vi "rpr -- read write buttons.vi"(7 "what":enum16{"read", "none", "write"}(ring)=enum."write", 8 "appended array":refnum<vi>[](array[refnum]), 9 "peaks":i32[](array[numeric])=[572], 11 "9w folder path":path=path "C:/data/RUS/Experiment/ProbeTest/Probe10/YBCO_6/sweep2/9w") -> ()   [LabVIEW 2014]
uses:
  <vilib>/Utility/file.llb/Read From Spreadsheet File (string).vi
  <vilib>/Utility/file.llb/Write To Spreadsheet File (string).vi
  <vilib>/regexp/Match Regular Expression.xnode
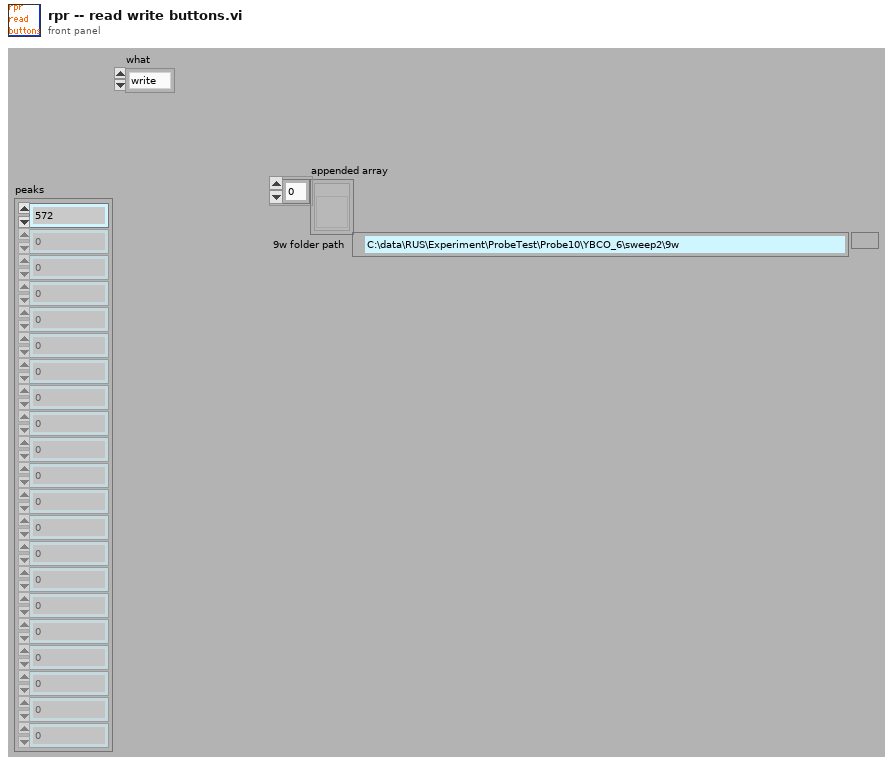
[diagram p1: front panel]
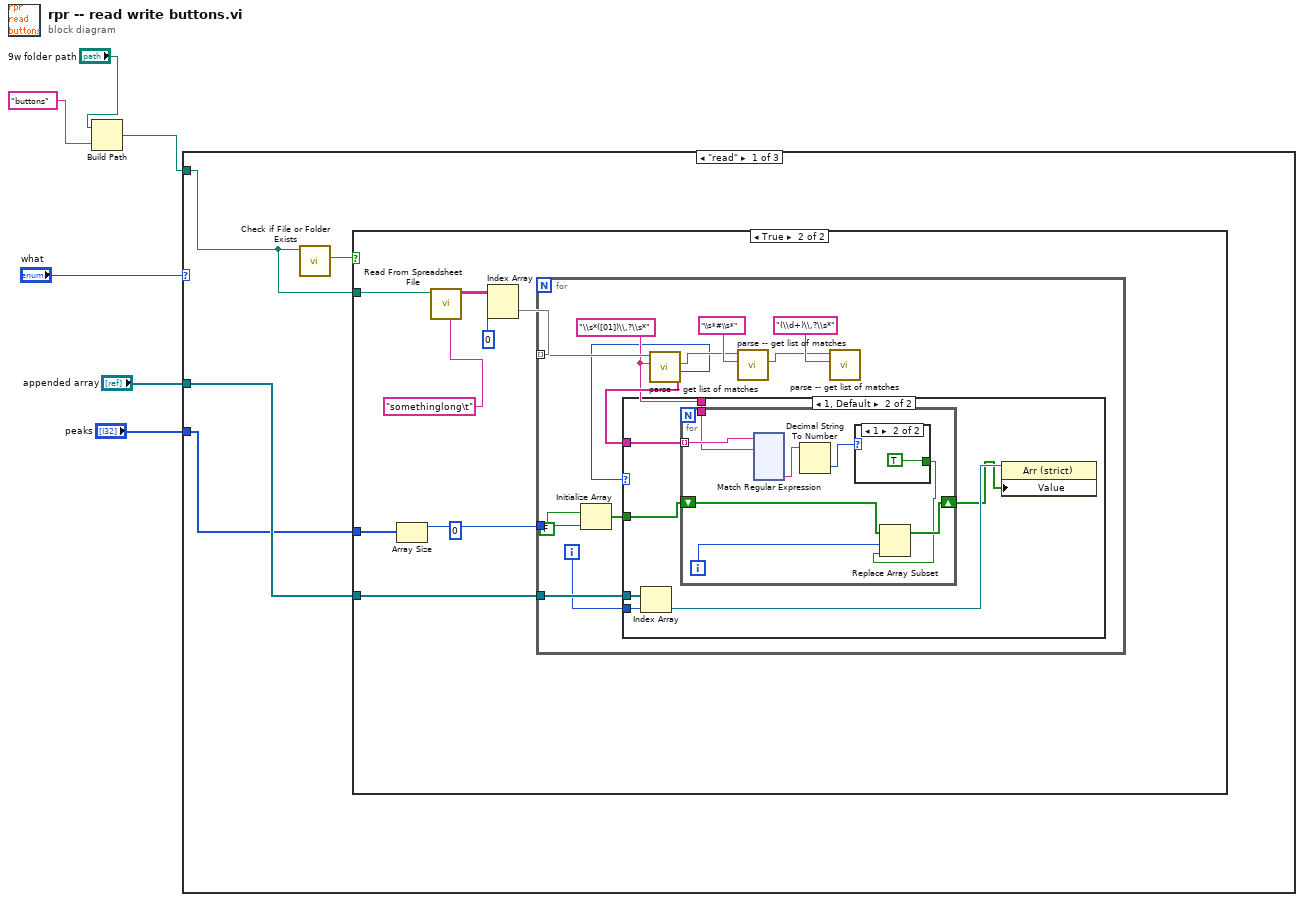
[diagram p0: block diagram]
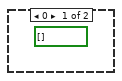
[diagram p3: hidden frame]
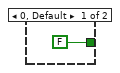
[diagram p4: hidden frame]
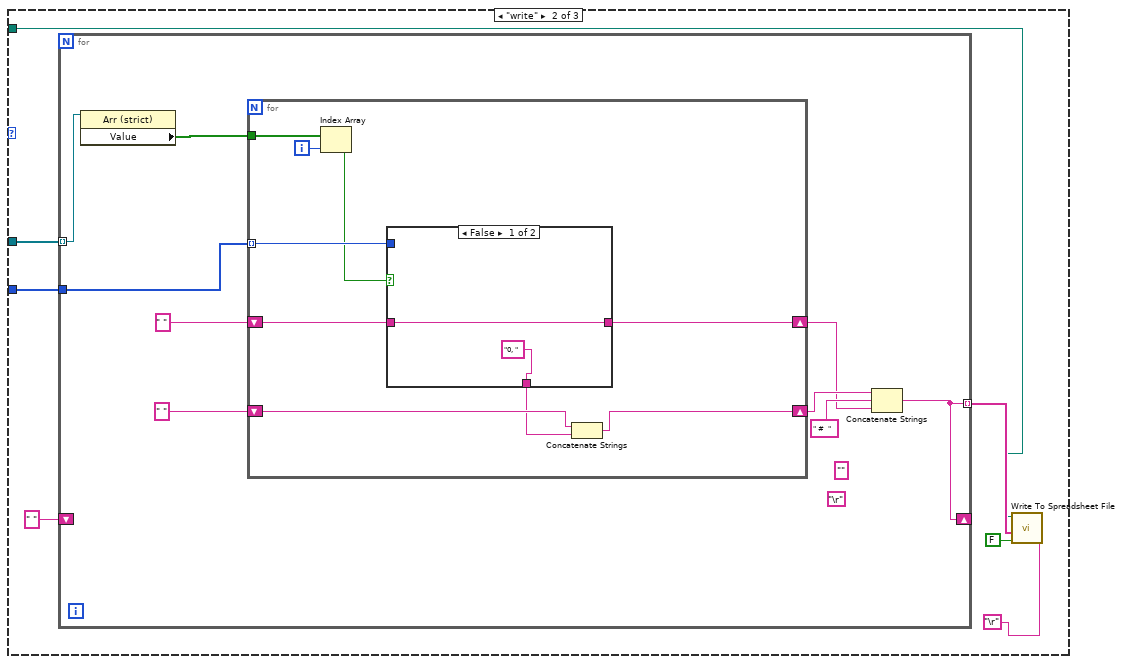
[diagram p5: hidden frame]
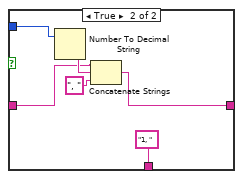
[diagram p6: hidden frame]
diagram:
  n1 = Build Path(base path="9w folder path", name or relative path="buttons") -> (appended path=w1:path)
  n2 = case shown="\"read\"" "what" {
    tunnel: "appended array" -> [w8 w168 _]
    tunnel: "peaks" -> [w7 w167 _]
    tunnel: w1 -> [w9 w162 _]
    frame "read" {
      n3 = call <vilib>:"Check if File or Folder Exists.vi"("path"=w9) -> ("file or folder exists?"=w10:bool)  [unwired: 8 in, 2 out]
      n4 = case shown="True" w10 {
        tunnel: w9 -> [_ w18]
        tunnel: w8 -> [_ w13]
        tunnel: w7 -> [_ w12]
        frame False {
        }
        frame True {
          (unwired) 0
          n5 = Array Size(array=w12) -> (size(s)=w11:i32)
          n6 = call-poly <vilib>:"Read From Spreadsheet File.vi"("delimiter (\\t)"="somethinglong\t" ("delimiter (\\t)"), "file path (dialog if empty)"=w18) -> ("all rows"=w16:string[][])  [unwired: 5 in, 4 out]
          n7 = Index Array(array=w16, index (col)=0) -> (element=w14:string[])  [unwired: 1 in]
          n8 = for {
            tunnel: w14 -> [w31] mode=indexing
            tunnel: w13 -> [w26]
            tunnel: w11 -> [w20]
            i -> [w25]
            w23 = "\\s*([01])\\,?\\s*" ("format string")
            n9 = Initialize Array(FALSE, w20) -> (w19:bool[])
            n10 = call "parse -- get list of matches.vi"("regexp"=w23, "string"=w31) -> ("Array"=w24:string[], "number of free elastic constants"=w22:i32, "after match"=w28:string)  [unwired: 7 in]
            n11 = case shown="1, Default" w22 {
              tunnel: w26 -> [_ w38]
              tunnel: w25 -> [_ w37]
              tunnel: w24 -> [_ w36]
              tunnel: w23 -> [_ w35]
              tunnel: w19 -> [_ w33]
              frame 0 {
                (unwired) bool[] []
              }
              frame 1, Default {
                n12 = Index Array(array=w38, index=w37) -> (element=w34:refnum<vi>)
                n13 = for {
                  tunnel: w36 -> [w46] mode=indexing
                  tunnel: w35 -> [w45]
                  shift-right: [w41] -> w32
                  shift-left: w33 -> [w42]
                  i -> [w40]
                  n14 = xnode "Match Regular Expression"("input string"=w46, "regular expression"=w45) -> ("submatch 1"=w44:string)  [unwired: 4 in, 5 out]
                  n15 = Decimal String To Number(string=w44) -> (number=w43:i32)  [unwired: 2 in, 1 out]
                  n16 = case shown="1" w43 {
                    tunnel: [FALSE TRUE] -> w39
                    frame 0, Default {
                    }
                    frame 1 {
                    }
                  }
                  n17 = Replace Array Subset(array=w42, new element=w39, index=w40) -> (w41:bool[])
                }
                n18 = property class="Arr (strict)"(reference=w34, "Value"=w32) -> ()  [unwired: 1 in, 2 out]
              }
            }
            n19 = call "parse -- get list of matches.vi"("regexp"="\\s*#\\s*" ("format string"), "string"=w28) -> ("after match"=w27:string)  [unwired: 7 in, 2 out]
            n20 = call "parse -- get list of matches.vi"("regexp"="(\\d+)\\,?\\s*" ("format string"), "string"=w27) -> ()  [unwired: 7 in, 3 out]
          }
        }
      }
    }
    frame "write" {
      n21 = for {
        tunnel: w168 -> [w177] mode=indexing
        tunnel: w167 -> [w175]
        shift-right: [w169] -> _
        shift-left: " " -> [_]
        tunnel: [w169] -> w165 mode=indexing
        (unwired) "\r"
        (unwired) ""
        n22 = property class="Arr (strict)"(reference=w177) -> ("Value"=w176:bool[])  [unwired: 1 in, 2 out]
        n23 = for {
          tunnel: w176 -> [w185]
          tunnel: w175 -> [w182] mode=indexing
          shift-right: [w183] -> w170
          shift-left: " " -> [w184]
          shift-right: [w178] -> w172
          shift-left: " " -> [w180]
          i -> [w186]
          n24 = Index Array(array=w185, index=w186) -> (element=w181:bool)
          n25 = case shown="False" w181 {
            tunnel: w184 -> [w188 w192]
            tunnel: [w188 w191] -> w183
            tunnel: w182 -> [_ w190]
            tunnel: ["0, " "1, "] -> w179
            frame False {
            }
            frame True {
              n26 = Number To Decimal String(number=w190) -> (decimal integer string=w194:string)  [unwired: 1 in]
              n27 = Concatenate Strings(w192, w194, ", ") -> (w191:string)
            }
          }
          n28 = Concatenate Strings(w180, w179) -> (w178:string)
        }
        n29 = Concatenate Strings(w172, " #  ", w170) -> (w169:string)
      }
      n30 = call-poly <vilib>:"Write To Spreadsheet File.vi"("delimiter (\\t)"="\r", "append to file? (new file:F)"=FALSE, "1D data"=w165, "file path (dialog if empty)"=w162) -> ()  [unwired: 4 in, 1 out]
    }
    frame "none", Default {
    }
  }
